vi "Read Configuration Data.vi"(8 "error in":errorcluster) -> (0 "error out":errorcluster, 3 "Configuration Data":T1)   [LabVIEW 2014]
uses:
  Configuration Data.ctl
  controls/MHL Configuration.ctl
  Controller/Controller Configuration.ctl
  Boiler/Boiler Configuration.ctl
  Boiler System Globals.vi
  <vilib>/Utility/config.llb/NI_LVConfig.lvlib
  Controller/Controller.lvlib
  Boiler/Boiler.lvlib
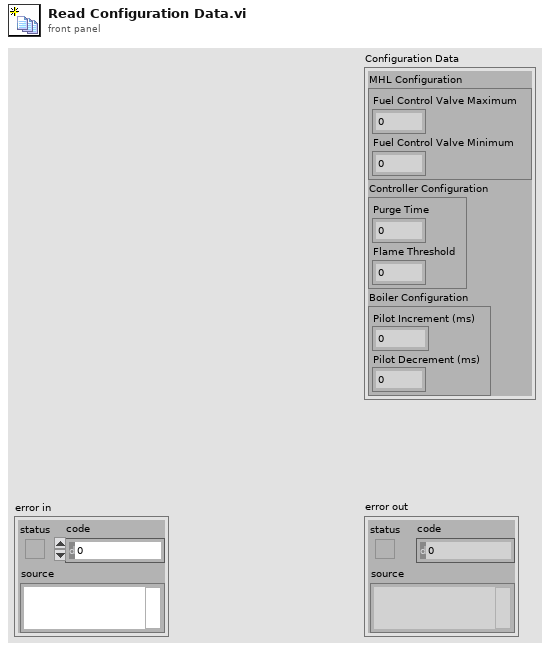
[diagram p1: front panel]
types:
  T1 = typedef "Configuration Data.ctl" = cluster{"MHL Configuration":T2, "Controller Configuration":T3, "Boiler Configuration":T4}
  T2 = typedef "MHL Configuration.ctl" = cluster{"Fuel Control Valve Maximum":dbl, "Fuel Control Valve Minimum":dbl}
  T3 = typedef "Controller.lvlib/Controller Configuration.ctl" = cluster{"Purge Time":u32, "Flame Threshold":u32}
  T4 = typedef "Boiler.lvlib/Boiler Configuration.ctl" = cluster{"Pilot Increment (ms)":u32, "Pilot Decrement (ms)":u32}
  T5 = enum32{"invalid app kind", "Development System", "Run Time System", "Student Edition", "Embedded LabVIEW", "Evaluation", "Custom"}
  T6 = typedef "NI_LVConfig.lvlib/Config Data RefNum.ctl" = refnum<k1>
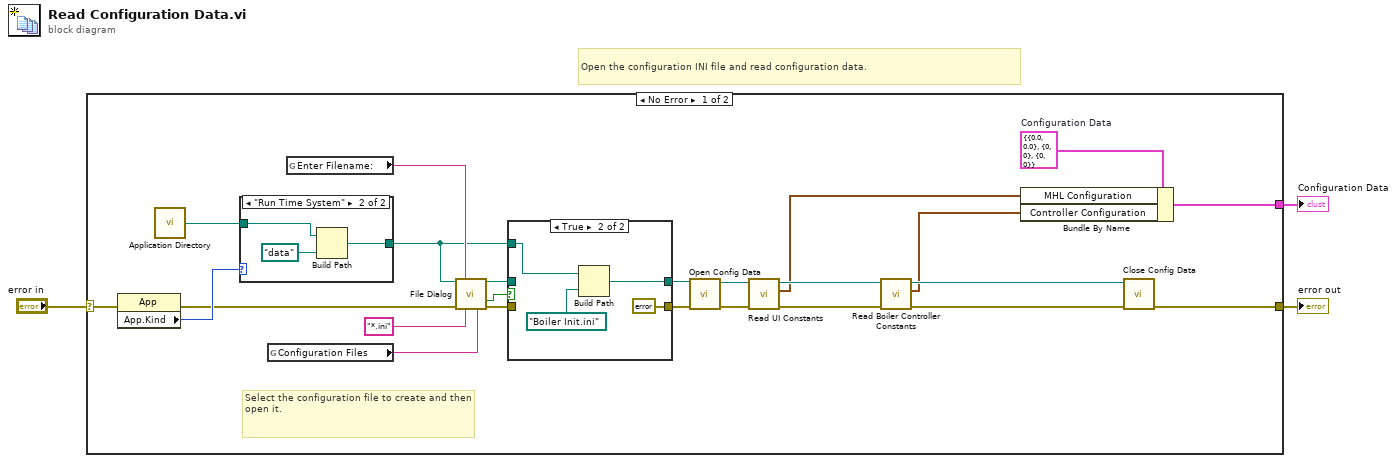
[diagram p0: block diagram]
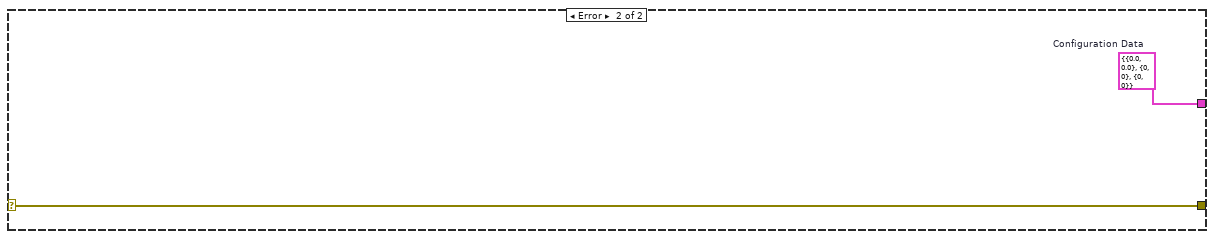
[diagram p4: hidden frame]
diagram:
  # "Open the configuration INI file and read configuration data."
  n1 = case shown="No Error" "error in" {
    selector: "error in" -> [w18 w39]
    tunnel: [w22 w39] -> w3
    tunnel: [w5 w38] -> w1
    frame No Error {
      w7 = T1 {"MHL Configuration"={"Fuel Control Valve Maximum"=0.0, "Fuel Control Valve Minimum"=0.0}, "Controller Configuration"={"Purge Time"=0, "Flame Threshold"=0}, "Boiler Configuration"={"Pilot Increment (ms)"=0, "Pilot Decrement (ms)"=0}}  # Configuration Data
      # "Select the configuration file to create and then open it."
      n2 = property class="App"(error in=w18) -> (error out=w17:errorcluster, "App.Kind"=w20:T5)  [unwired: 1 in, 1 out]
      n3 = call <vilib>:"Application Directory.vi"() -> ("Application Directory"=w19:path)
      n4 = case shown="\"Run Time System\"" w20 {
        tunnel: w19 -> [w34 w37]
        tunnel: [w34 w35] -> w11
        frame Default {
        }
        frame "Run Time System" {
          n5 = Build Path(base path=w37, name or relative path=path "data") -> (appended path=w35:path)
        }
      }
      n6 = global read "Boiler System Globals.vi" "Configuration Files"() -> (w25:string)
      n7 = global read "Boiler System Globals.vi" "Enter Filename:"() -> (w27:string)
      n8 = call "File Dialog"("start path"=w11, "prompt"=w27, "error in"=w17, "pattern (all files)"="*.ini", "pattern label"=w25) -> ("selected path"=w14:path, "cancelled"=w16:bool, "error out"=w15:errorcluster)  [unwired: 7 in, 1 out]
      n9 = case shown="True" w16 {
        tunnel: w15 -> [w29 _]
        tunnel: w14 -> [w28 _]
        tunnel: [w29 errorcluster {"status"=FALSE, "code"=0, "source"=""} ("error out")] -> w13
        tunnel: [w28 w32] -> w12
        tunnel: w11 -> [_ w33]
        frame False {
        }
        frame True {
          n10 = Build Path(base path=w33, name or relative path=path "Boiler Init.ini") -> (appended path=w32:path)
        }
      }
      n11 = call <vilib>:"Open Config Data.vi"("error in (no error)"=w13, "configuration file path"=w12) -> ("error out"=w23:errorcluster, "refnum"=w24:T6)  [unwired: 1 in, 7 out]
      n12 = call "Read UI Constants.vi"("error in"=w23, "CFG File Refnum in"=w24) -> ("error out"=w21:errorcluster, "MHL Configuration"=w6:T2, "CFG File Refnum out"=w9:T6)  [unwired: 7 in]
      n13 = call "Read Boiler Controller Constants.vi"("error in"=w21, "CFG File Refnum in"=w9) -> ("error out"=w10:errorcluster, "Controller Configuration"=w4:T3, "CFG File Refnum out"=w8:T6)  [unwired: 7 in]
      n14 = Bundle By Name(cluster=w7, "MHL Configuration"=w6, "Controller Configuration"=w4) -> (w5:T1)
      n15 = call <vilib>:"Close Config Data.vi"("error in (no error)"=w10, "refnum"=w8) -> ("error out"=w22:errorcluster)  [unwired: 1 in, 8 out]
    }
    frame Error {
      w38 = T1 {"MHL Configuration"={"Fuel Control Valve Maximum"=0.0, "Fuel Control Valve Minimum"=0.0}, "Controller Configuration"={"Purge Time"=0, "Flame Threshold"=0}, "Boiler Configuration"={"Pilot Increment (ms)"=0, "Pilot Decrement (ms)"=0}}  # Configuration Data
    }
  }
  "error out" <- w3
  "Configuration Data" <- w1
